vi "VI_FP close.vi"(8 "error in (no error)":errorcluster, 11 "VI in":refnum<vi>) -> (0 "error out":errorcluster, 3 "VI out":refnum<vi>)   [LabVIEW 2015]
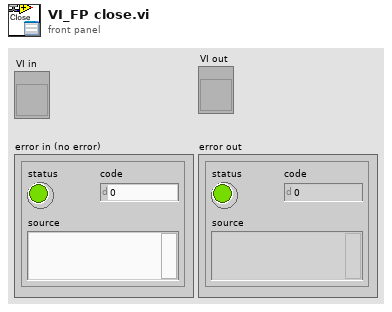
[diagram p1: front panel]
types:
  T1 = enum32{"invalid app kind", "Development System", "Run Time System", "Student Edition", "Embedded LabVIEW", "Evaluation", "Custom"}
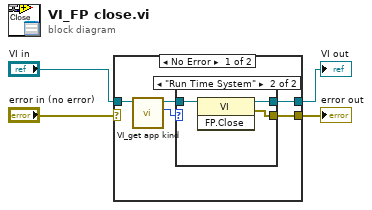
[diagram p0: block diagram]
diagram:
  n1 = case shown="No Error" "error in (no error)" {
    selector: "error in (no error)" -> [_ w14]
    tunnel: [w9 w15] -> w4
    tunnel: "VI in" -> [w7 w15]
    tunnel: [w8 w14] -> w1
    frame No Error {
      n2 = call "VI_get app kind.vi"("VI in"=w7) -> ("App.Kind"=w5:T1, "VI out"=w6:refnum<vi>)  [unwired: 8 in, 1 out]
      n3 = case shown="\"Run Time System\"" w5 {
        tunnel: [w10 w13] -> w9
        tunnel: [_ w12] -> w8
        tunnel: w6 -> [w10 w11]
        frame Default {
        }
        frame "Run Time System" {
          n4 = invoke class="VI" method="FP.Close"(reference=w11) -> (reference out=w13:refnum<vi>, error out=w12:errorcluster)  [unwired: 2 in, 1 out]
        }
      }
    }
    frame Error {
    }
  }
  "VI out" <- w4
  "error out" <- w1
